vi "CLD 8 CSV file commands utility Solution.vi"(8 "Error In":errorcluster) -> (0 "Error Out":errorcluster, 3 "Commands Out Array":T1[](array[typedef]))   [LabVIEW 2018]
doc: "CLD 8: Reads data from CSV and inserts into array of clusters."
uses:
  CLD 8 Data Cluster.ctl
  <vilib>/Utility/file.llb/Read Delimited Spreadsheet (string).vi
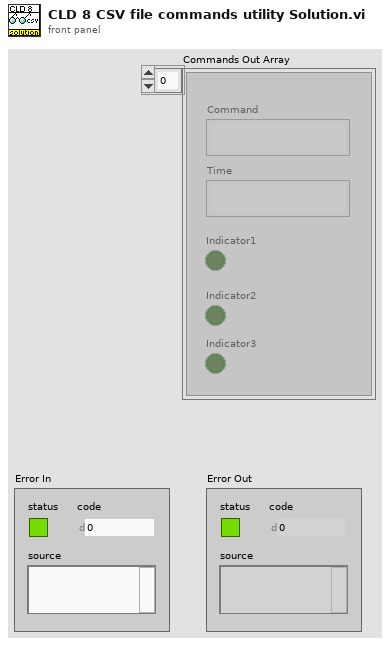
[diagram p1: front panel]
types:
  T1 = typedef "CLD 8 Data Cluster.ctl" = cluster{"Command":string, "Time":string, "Indicator1":bool, "Indicator2":bool, "Indicator3":bool}
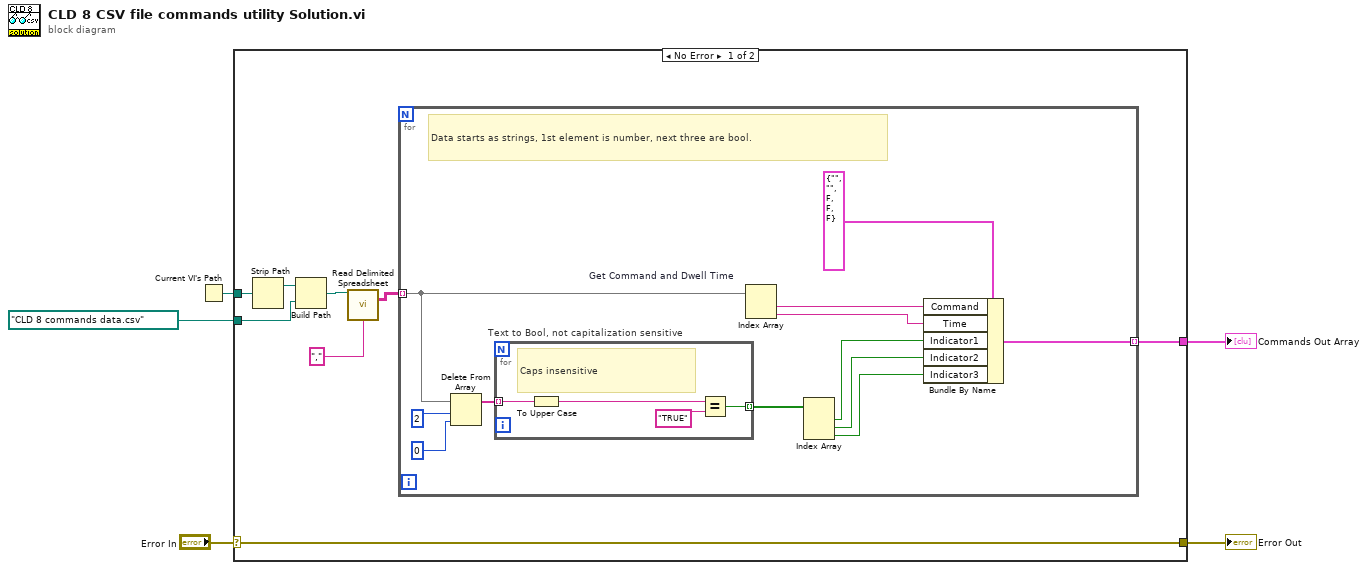
[diagram p0: block diagram]
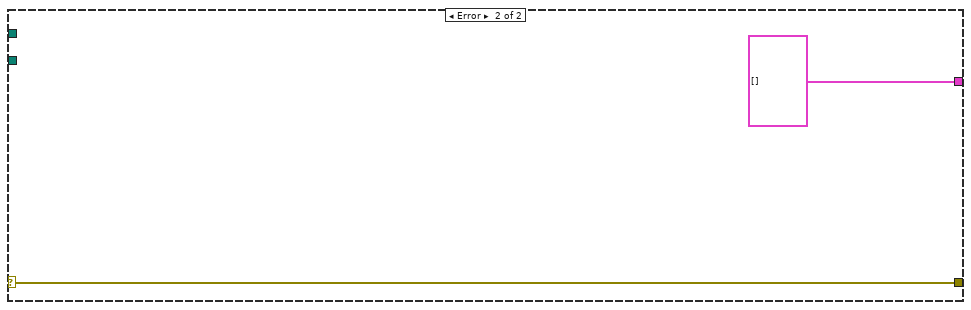
[diagram p2: hidden frame]
diagram:
  n1 = Current VI's Path() -> (path=w2:path)
  n2 = case shown="No Error" "Error In" {
    selector: "Error In" -> [w13 w31]
    tunnel: [w11 T1[] []] -> w1
    tunnel: path "CLD 8 commands data.csv" -> [w9 _]
    tunnel: w2 -> [w10 _]
    tunnel: [w13 w31] -> w3
    frame No Error {
      n3 = Strip Path(path=w10) -> (stripped path=w7:path)  [unwired: 1 out]
      n4 = Build Path(base path=w7, name or relative path=w9) -> (appended path=w8:path)
      n5 = call-poly <vilib>:"Read Delimited Spreadsheet.vi"("file path (dialog if empty)"=w8, "delimiter (\\t)"="," ("delimiter (\\t)")) -> ("all rows"=w6:string[][])  [unwired: 8 in, 5 out]
      n6 = for {
        tunnel: w6 -> [w25] mode=indexing
        tunnel: [w14] -> w11 mode=indexing
        # "Data starts as strings, 1st element is number, next three are bool."
        n7 = Delete From Array(array=w25, length=2, index=0) -> (array with subset deleted=w21:string[])  [unwired: 1 out]
        n8 = for "Text to Bool, not capitalization sensitive" {
          tunnel: w21 -> [w29] mode=indexing
          tunnel: [w26] -> w22 mode=indexing
          # "Caps insensitive"
          n9 = To Upper Case(1:w29) -> (0:w28:string)
          n10 = Equal?(x=w28, y="TRUE") -> (x = y?=w26:bool)
        }
        n11 = Index Array "Get Command and Dwell Time"(array=w25) -> (element #1=w19:string, element #2=w18:string)  [unwired: 2 in]
        n12 = Index Array(array=w22) -> (element #1=w17:bool, element #2=w16:bool, element #3=w15:bool)  [unwired: 3 in]
        n13 = Bundle By Name(cluster=T1 {"Command"="", "Time"="", "Indicator1"=FALSE, "Indicator2"=FALSE, "Indicator3"=FALSE} ("Cluster 3"), "Command"=w19, "Time"=w18, "Indicator1"=w17, "Indicator2"=w16, "Indicator3"=w15) -> (w14:T1)
      }
    }
    frame Error {
    }
  }
  "Error Out" <- w3
  "Commands Out Array" <- w1
